vi "GUI_LP_Mode_Filter.vi"() -> ()   [LabVIEW 2020]
uses:
  Shared/GUI_Template/GUI_master/tcp_new_data_event.ctl
  Shared/GUI_Template/GUI_master/tcp new data cluster.ctl
panel:
  in  "RetractPosition.Channel 5::1":dbl caption="Set OFF Position (OD4-CH5)" min=0.0 max=52.0
  in  "RetractPosition.Channel 3::1":dbl caption="Set OFF Position (LPMode-CH3)" min=0.0 max=80.0
  in  "RetractPosition.Channel 4::1":dbl caption="Set OFF Position (OD2-CH4)" min=0.0 max=52.0
  in  "RetractPosition.Channel 2::1":dbl caption="Set OFF Position (OD3-CH2)" min=0.0 max=52.0
  in  "RetractPosition.Channel 1::1":dbl caption="Set OFF Position (OD1-CH1)" min=0.0 max=52.0
  in  "ReferencePosition.Channel 1::1":dbl caption="Set Current Position as...(OD1-CH1)" min=0.0 max=52.0
  in  "ExtendPosition.Channel 5::1":dbl caption="Set ON Position (OD4-CH5)" min=0.0 max=52.0
  in  "ReferencePosition.Channel 5::1":dbl caption="Set Current Position as...(OD4-CH5)" min=0.0 max=52.0
  in  "Position.Channel 5::1":dbl caption="Position OD4 (CH5)" min=0.0 max=52.0 format="%#_6p"
  in  "filter.Channel 5::1":enum16{"off", "on"}(ring) caption="OD4 (CH5)"
  in  "Resize Button":bool
  in  "ExtendPosition.Channel 3::1":dbl caption="Set Extend Position (LPMode-CH3)" min=0.0 max=80.0
  in  "ExtendPosition.Channel 4::1":dbl caption="Set ON Position (OD2-CH4)" min=0.0 max=52.0
  in  "ExtendPosition.Channel 2::1":dbl caption="Set ON Position (OD3-CH2)" min=0.0 max=52.0
  in  "ExtendPosition.Channel 1::1":dbl caption="Set ON Position (OD1-CH1)" min=0.0 max=52.0
  in  "ReferencePosition.Channel 3::1":dbl caption="Set Current Position as...(LPMode-CH3)" min=0.0 max=82.0
  in  "Position.Channel 4::1":dbl caption="Position OD2 (CH4)" min=0.0 max=52.0 format="%#_6p"
  in  "Position.Channel 3::1":dbl caption="Position (LP Mode)" min=0.0 max=70.0 format="%#_6p"
  in  "Position.Channel 2::1":dbl caption="Position OD3 (CH2)" min=0.0 max=52.0 format="%#_6p"
  in  "Position.Channel 1::1":dbl caption="Position OD1 (CH1)" min=-25.0 max=52.0 format="%#_6p"
  in  "ReferencePosition.Channel 4::1":dbl caption="Set Current Position as...(OD2-CH4)" min=0.0 max=52.0
  in  "ReferencePosition.Channel 2::1":dbl caption="Set Current Position as...(OD3-CH2)" min=0.0 max=52.0
  in  "filter.Channel 4::1":enum16{"off", "on"}(ring) caption="OD2 (CH4)"
  in  "filter.Channel 2::1":enum16{"off", "on"}(ring) caption="OD3 (CH2)"
  in  "filter.Channel 1::1":enum16{"off", "on"}(ring) caption="OD1 (CH1)"
  in  "insert tag":bool=TRUE
  in  "stop":bool
  in  "GUIdevice 1":string="STAGE-PL1-Smaract"
  out "tcp data event":T1
  out "error IO 2":errorcluster
  # "LP MODE FILTERS and CAM STAGES"
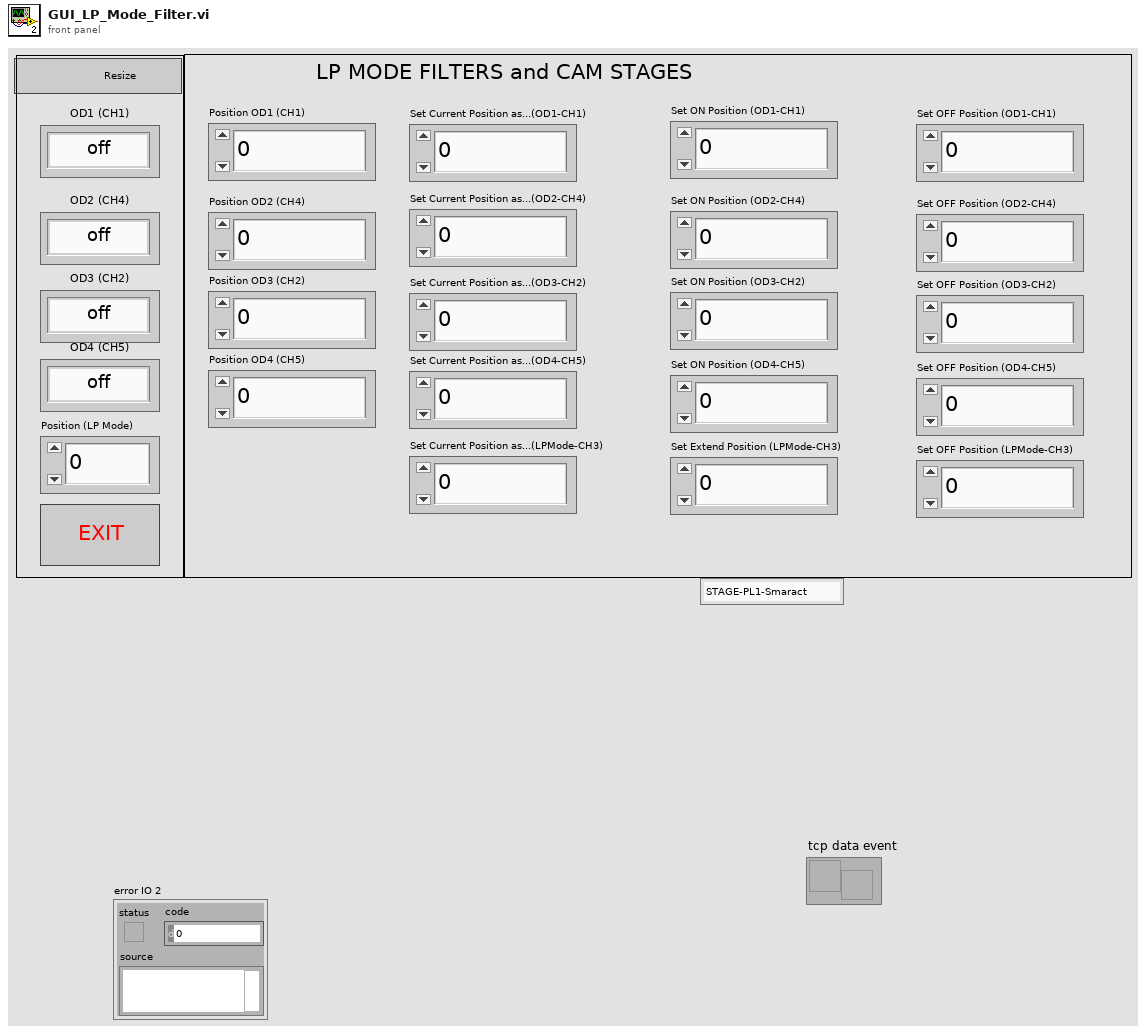
[diagram p1: front panel]
types:
  T1 = typedef "tcp_new_data_event.ctl" = refnum<user-event>
  T2 = typedef "tcp new data cluster.ctl" = cluster{"EventEnum":enum16{"new data", "connection status update"}, "Device name":string}
  T3 = typedef "LVRectTypeDef.ctl" = cluster{"Left":i16, "Top":i16, "Right":i16, "Bottom":i16}
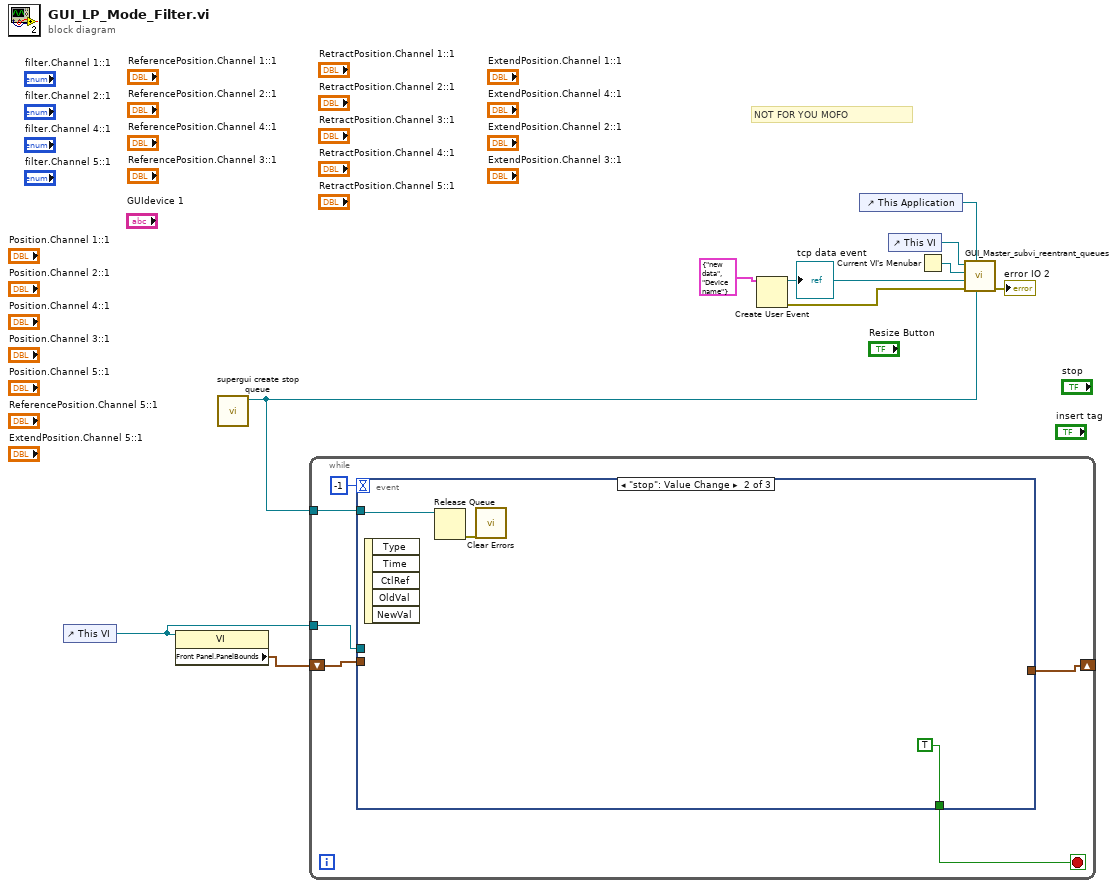
[diagram p0: block diagram]
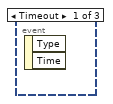
[diagram p2: hidden frame]
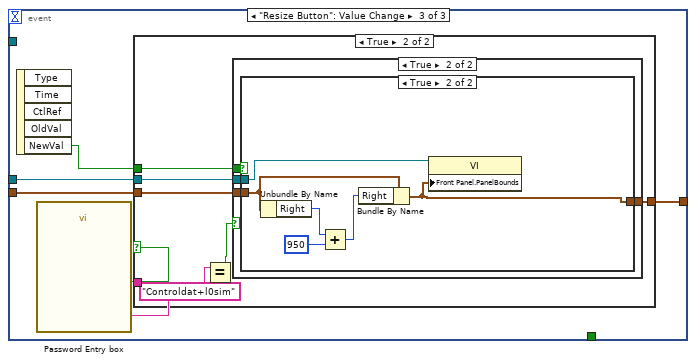
[diagram p3: hidden frame]
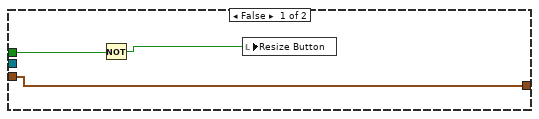
[diagram p4: hidden frame]
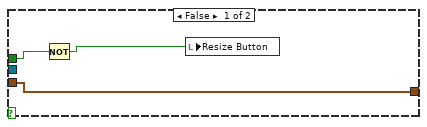
[diagram p5: hidden frame]
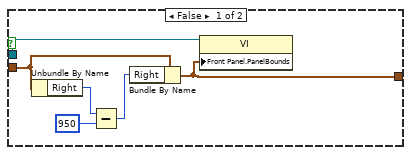
[diagram p6: hidden frame]
diagram:
  # "NOT FOR YOU MOFO"
  n1 = control-ref of="This VI"() -> (w3:refnum<vi>)
  n2 = property class="VI"(reference=w3) -> ("Front Panel.PanelBounds"=w4:T3)  [unwired: 1 in, 2 out]
  n3 = call "supergui create stop queue.vi"() -> ("STOP Queue out"=w1:refnum<queue>)  [unwired: 11 in]
  n4 = while {
    shift-right: [w12] -> _
    shift-left: w4 -> [w13]
    tunnel: w3 -> [w14]
    tunnel: w1 -> [w11]
    stop <- w15 stop-if-true
    n5 = event shown="[1] \"stop\": Value Change" {
      selector: _ -> [_ _ _]
      dyn-events: _ -> [_ _ _]
      timeout: -1 -> [_ _ _]
      tunnel: [_ TRUE _] -> w15
      tunnel: w14 -> [_ _ w24]
      tunnel: w13 -> [_ _ w23]
      tunnel: [_ _ w22] -> w12
      tunnel: w11 -> [_ w18 _]
      event Timeout {
        n6 = event-data() -> ()  [unwired: 1 in, 2 out]
      }
      event "stop": Value Change {
        n7 = event-data() -> ()  [unwired: 1 in, 5 out]
        n8 = Release Queue(queue=w18) -> (error out=w17:errorcluster)  [unwired: 2 in, 2 out]
        n9 = call <vilib>:"Clear Errors.vi"("error in (no error)"=w17) -> ()  [unwired: 5 in, 2 out]
      }
      event "Resize Button": Value Change {
        n10 = event-data() -> ("NewVal"=w25:bool)  [unwired: 1 in, 4 out]
        n11 = call "Password Entry box.vi"() -> ("Password"=w20:string, "OK"=w21:bool)  [unwired: 17 in, 1 out]
        n12 = case shown="True" w21 {
          tunnel: w25 -> [w27 w35]
          tunnel: w24 -> [_ w34]
          tunnel: w23 -> [w28 w33]
          tunnel: [w28 w32] -> w22
          tunnel: w20 -> [_ w31]
          frame False {
            n13 = Not(x=w27) -> (.not. x?=w26:bool)
            n14 = local write "Resize Button"(w26) -> ()
          }
          frame True {
            n15 = Equal?(x=w31, y="Controldat+l0sim") -> (x = y?=w29:bool)
            n16 = case shown="True" w29 {
              tunnel: w35 -> [w36 w42]
              tunnel: w34 -> [_ w41]
              tunnel: w33 -> [w38 w40]
              tunnel: [w38 w39] -> w32
              frame False {
                n17 = Not(x=w36) -> (.not. x?=w37:bool)
                n18 = local write "Resize Button"(w37) -> ()
              }
              frame True {
                n19 = case shown="True" w42 {
                  tunnel: w41 -> [w48 w52]
                  tunnel: w40 -> [w47 w51]
                  tunnel: [w43 w50] -> w39
                  frame False {
                    n20 = Unbundle By Name(w47) -> ("Right"=w46:i16)
                    n21 = Subtract(x=w46, y=i16 950) -> (x-y=w44:i16)
                    n22 = Bundle By Name(cluster=w47, "Right"=w44) -> (w43:T3)
                    n23 = property class="VI"(reference=w48, "Front Panel.PanelBounds"=w43) -> ()  [unwired: 1 in, 2 out]
                  }
                  frame True {
                    n24 = Unbundle By Name(w51) -> ("Right"=w54:i16)
                    n25 = Add(x=w54, y=i16 950) -> (x+y=w53:i16)
                    n26 = Bundle By Name(cluster=w51, "Right"=w53) -> (w50:T3)
                    n27 = property class="VI"(reference=w52, "Front Panel.PanelBounds"=w50) -> ()  [unwired: 1 in, 2 out]
                  }
                }
              }
            }
          }
        }
      }
    }
  }
  n28 = Create User Event(user event datatype=T2 {"EventEnum"=enum."new data", "Device name"="Device name"} ("New Event")) -> (user event=w5:refnum<user-event>, error out=w6:errorcluster)  [unwired: 1 in]
  "tcp data event" <- w5
  n29 = control-ref of="This Application"() -> (w2:refnum<vi>)
  n30 = control-ref of="This VI"() -> (w9:refnum<vi>)
  n31 = Current VI's Menubar() -> (w8:refnum<k9>)
  n32 = call "GUI_Master_subvi_reentrant_queues.vi"("STOP Queue in"=w1, "This Application"=w2, "error in (no error)"=w6, "tcp data event"=w5, "Caller menu reference"=w8, "Caller VI ref"=w9) -> ("error out"=→"error IO 2":errorcluster)  [unwired: 5 in]
